vi "cont_acquisition.vi"() -> ()   [LabVIEW 2011]
uses:
  global_vars.vi
  <vilib>/vision/driver/NI_Vision_Acquisition_Software.lvlib
panel:
  in  "Color":u32(colorbox)=16448250
  in  "center radius":dbl
  in  "number of rings":i32
  out "Frame Rate":dbl
  in  "Close":bool
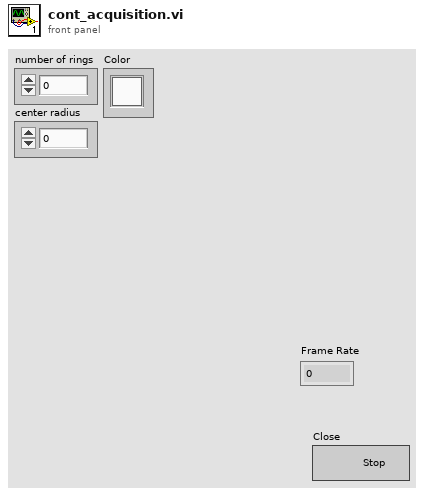
[diagram p1: front panel]
types:
  T1 = typedef "IMAQdx.ctl" = refnum<k21>
  T2 = typedef "IMAQ Image.ctl" = refnum<image>
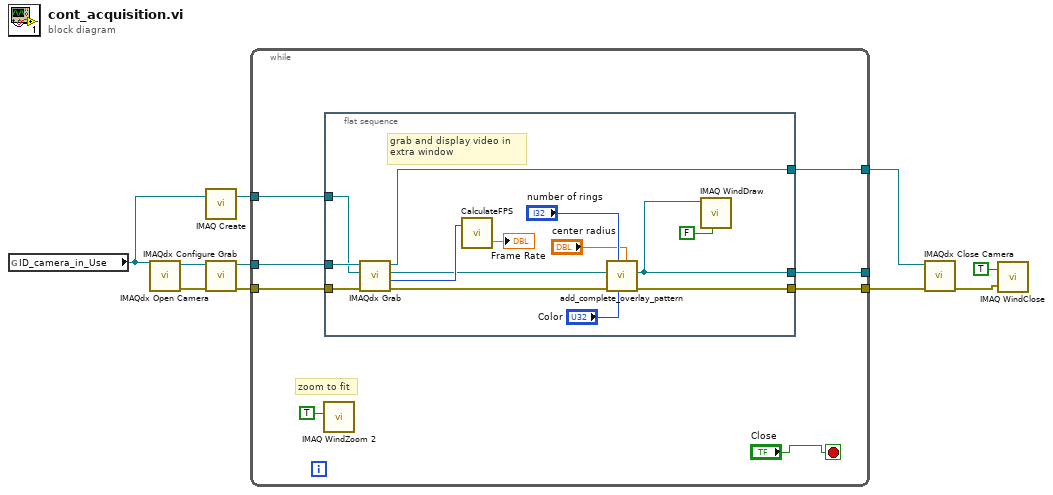
[diagram p0: block diagram]
diagram:
  n1 = global read "global_vars.vi" "ID_camera_in_Use"() -> (w2:T1)
  n2 = call <vilib>:"IMAQdx Open Camera.vi"("Session In"=w2) -> ("error out"=w6:errorcluster, "Session Out"=w5:T1)  [unwired: 2 in, 7 out]
  n3 = call "IMAQ Create"("Image Name"=w2) -> ("New Image"=w10:T2)  [unwired: 3 in, 2 out]
  n4 = call <vilib>:"IMAQdx Configure Grab.vi"("error in"=w6, "Session In"=w5) -> ("error out"=w8:errorcluster, "Session Out"=w9:T1)  [unwired: 8 out]
  n5 = while {
    tunnel: w8 -> [w17]
    tunnel: w9 -> [w18]
    tunnel: [w15] -> w7
    tunnel: w10 -> [w16]
    tunnel: [w13] -> _
    tunnel: [w12] -> w1
    stop <- "Close" stop-if-true
    # "zoom to fit"
    n6 = call "IMAQ WindZoom 2"("Zoom to Fit? (False)"=TRUE) -> ()  [unwired: 7 in, 4 out]
    n7 = flat-sequence {
      tunnel: [w28] -> w15
      tunnel: w18 -> [w31]
      tunnel: w17 -> [w30]
      tunnel: w16 -> [w29]
      tunnel: [w20] -> w13
      tunnel: [w19] -> w12
      frame #0 {
        # "grab and display video in \nextra window"
        n8 = call <vilib>:"IMAQdx Grab.vi"("error in"=w30, "Image In"=w29, "Session In"=w31) -> ("error out"=w28:errorcluster, "Buffer Number Out"=w26:u32, "Image Out"=w24:T2, "Session Out"=w19:T1)  [unwired: 1 in, 4 out]
        n9 = call "CalculateFPS.vi"("buffer number"=w26) -> ("processed FPS"=→"Frame Rate":dbl)  [unwired: 2 out]
        n10 = call "add_complete_overlay_pattern.vi"("center radius"="center radius", "Color"="Color", "number of rings"="number of rings", "Image Src"=w24) -> ("Image Out"=w20:T2)  [unwired: 7 in]
        n11 = call "IMAQ WindDraw"("Resize to Image Size? (Y)"=FALSE, "Image"=w20) -> ()  [unwired: 8 in, 2 out]
      }
    }
  }
  n12 = call <vilib>:"IMAQdx Close Camera.vi"("error in"=w7, "Session In"=w1) -> ("error out"=w3:errorcluster)  [unwired: 9 out]
  n13 = call "IMAQ WindClose"("Close All Windows (False)"=TRUE, "error in (no error)"=w3) -> ()  [unwired: 4 in, 1 out]
